vi "create.vi"(8 "error in":errorcluster, 10 "max queue size (50)":i32=50) -> (0 "error out":errorcluster, 3 "stream publisher out":refnum<class "subscriber.lvclass">)   [LabVIEW 2013, in "data stream.lvlib" / "subscriber.lvclass"]
uses:
  subscriber.lvclass
  stream definition.ctl
  message definition.ctl
  subscriber.lvclass/subscriber.ctl
  data stream.lvlib
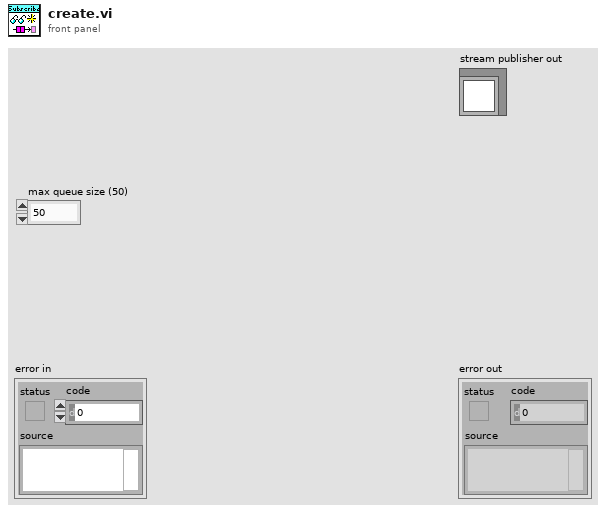
[diagram p1: front panel]
types:
  T1 = typedef "data stream.lvlib/stream definition.ctl" = cluster{"contained data":T2, "message name":string, "Waveform":waveform(dbl), "payload":variant}
  T2 = typedef "data stream.lvlib/message definition.ctl" = enum16{"waveform", "message"}
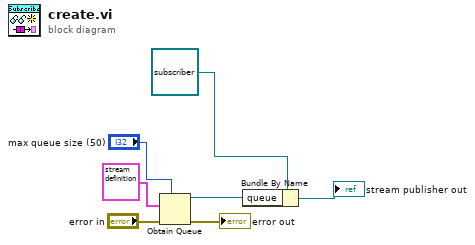
[diagram p0: block diagram]
diagram:
  n1 = Obtain Queue(max queue size (-1, unlimited)="max queue size (50)", element data type=T1 {"contained data"=enum."waveform", "message name"="", "Waveform"={"t0"=timestamp(0 s since 1904-01-01), "dt"=1.0, "Y"=[]}, "payload"=variant} ("stream definition"), error in (no error)="error in") -> (queue out=w1:refnum<queue>, error out=→"error out":errorcluster)  [unwired: 2 in, 1 out]
  n2 = Bundle By Name(cluster=refnum<class "subscriber.lvclass"> refnum ("stream publisher in"), "queue"=w1) -> (→"stream publisher out":refnum<class "subscriber.lvclass">)
